vi "Simultaneous generation of analog voltage and digital signals.vi"() -> ()   [LabVIEW 2023]
uses:
  <vilib>/Utility/error.llb/DialogType.ctl
  <vilib>/DAQmx/configure/timing.llb/DAQmx Timing (Sample Clock).vi
  <vilib>/DAQmx/miscellaneous.llb/DAQmx Fill In Error Info.vi
  <vilib>/Waveform/DWDTOps.llb/DWDT Uncompress Digital.vi
  <vilib>/DAQmx/configure/trigger.llb/DAQmx Start Trigger (Digital Edge).vi
  <vilib>/DAQmx/create/channels.llb/DAQmx Create Channel (CO-Pulse Generation-Time).vi
  <vilib>/DAQmx/write.llb/DAQmx Write (Digital 1D Wfm NChan NSamp).vi
  <vilib>/DAQmx/create/channels.llb/DAQmx Create Channel (DO-Digital Output).vi
  <vilib>/DAQmx/write.llb/DAQmx Write (Analog 1D Wfm NChan NSamp).vi
  <vilib>/Waveform/DWDTOps.llb/DWDT Analog to Digital.vi
  <vilib>/DAQmx/create/channels.llb/DAQmx Create Channel (AO-Voltage-Basic).vi
  <resource>/objmgr/daqmx.rc
  <vilib>/measure/NI_MABase.lvlib
panel:
  in  "% of the time LEDs are shining\n(100 % maximum)":u32
  in  "Digital Channels for trigerring":tag
  out "Digital Waveform Graph":digitalwaveform[](graph)
  out "Waveform Graph":waveform(dbl)[](graph)
  in  "Stop Generation":bool caption="Stop Waveform Generation"
  in  "Analog Output Channels":tag
  out "Actual Duty Cycle (%)":dbl
  in  "Duty Cycle (%)":dbl
  in  "Square Wave Frequency (Hz)":dbl
  in  "LED Bias Voltage (V)":dbl[](array[numeric])
  # "AO0"
  # "AO1"
  # "AO2"
  # "AO3"
  # "If the duty cycle is set to 0, the default duty cycle will be applied, which depends on the number of channels active. 2 channels -> 50 %, 3 channels -> 33.33 %, 4 channels -> 25 %."
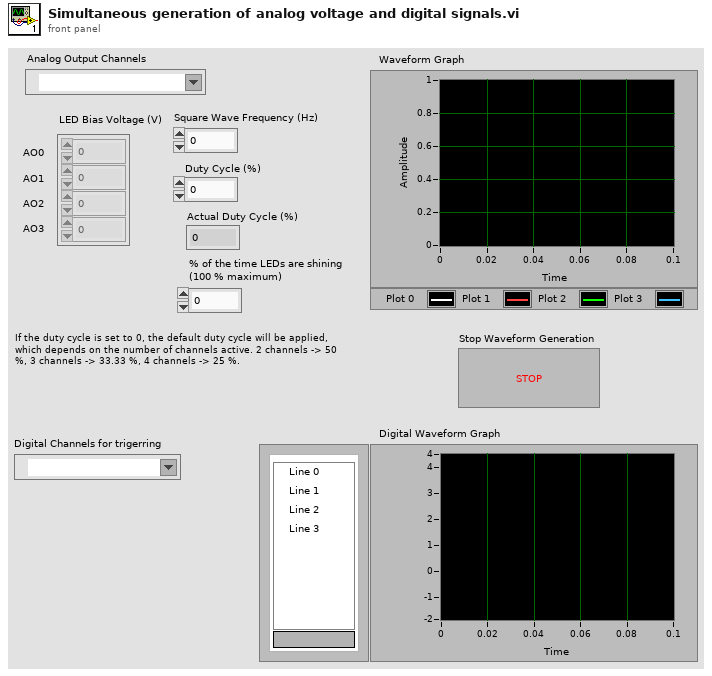
[diagram p1: front panel]
types:
  T1 = typedef "DialogType.ctl" = u16
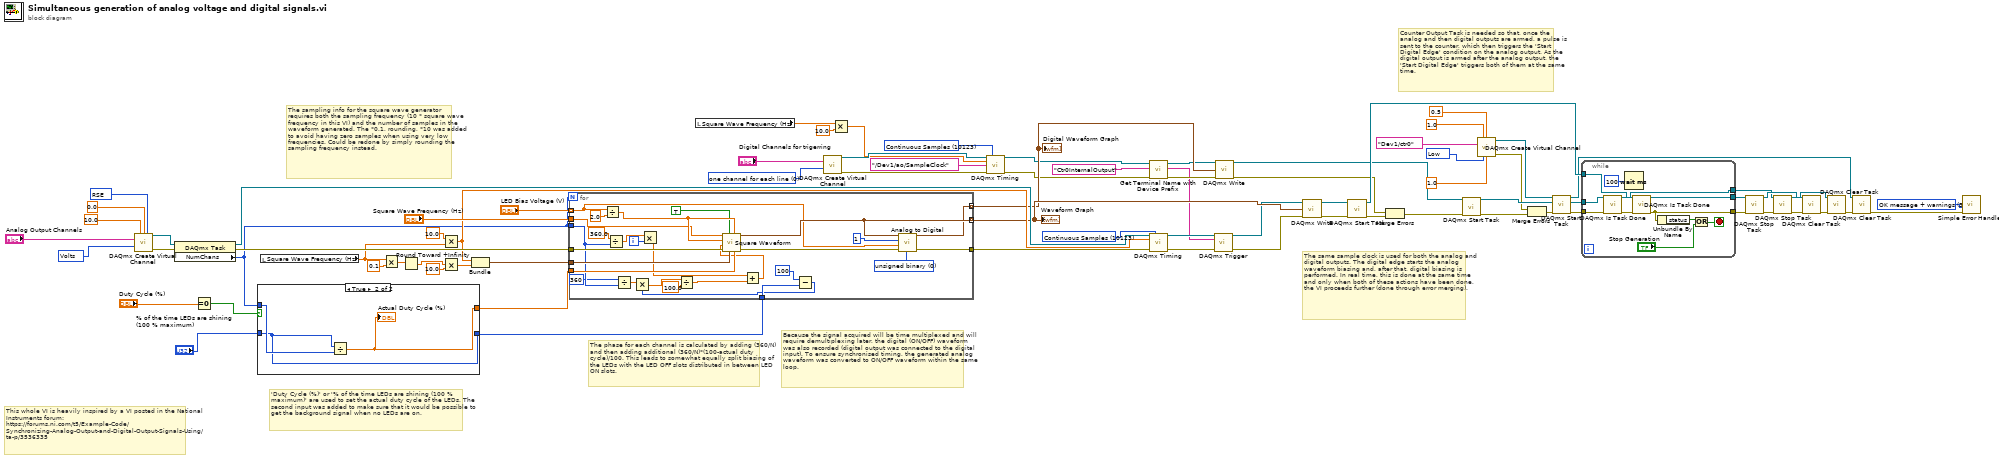
[diagram p0: block diagram]
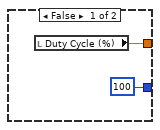
[diagram p2: hidden frame]
diagram:
  w24 = 10214 items=["High"=10192, "Low"=10214] ("idle state")
  w28 = 0 items=["one channel for each line", "one channel for all lines"] ("line grouping")
  w46 = 10123 items=["Finite Samples"=10178, "Continuous Samples"=10123, "Hardware Timed Single Point"=12522] ("sample mode")
  w52 = T1 3 items=["no dialog", "OK message", "continue or stop message", "OK message + warnings", "continue/stop + warnings"] ("type of dialog (OK msg:1)")
  w60 = 10123 items=["Finite Samples"=10178, "Continuous Samples"=10123, "Hardware Timed Single Point"=12522] ("sample mode")
  w77 = 10083 items=["Default"=-1, "RSE"=10083, "Differential"=10106, "Pseudodifferential"=12529] ("output terminal configuration")
  w78 = 10348 items=["Volts"=10348, "From Custom Scale"=10065] ("units")
  # "This whole VI is heavily inspired by a VI posted in the National Instruments forum:\nhttps://forums.ni.com/t5/Example-Code/Synchronizing-Analog-Output-and-Digital-Output-Signals-Using/ta-p/3536335"
  # "Counter Output Task is needed so that, once the analog and then digital outputs are armed, a pulse is sent to the counter, which then triggers the 'Start Digital Edge' condition on the analog output. As the digital output is armed after the analog output, the 'Start Digital Edge' triggers both of them at the same time."
  # "The same sample clock is used for both the analog and digital outputs. The digital edge starts the analog waveform biasing and, after that, digital biasing is performed. In real time, this is done at the same time and only when both of these actions have been done, the VI proceeds further (done through error merging)."
  # "Because the signal acquired will be time multiplexed and will require demultiplexing later, the digital (ON/OFF) waveform was also recorded (digital output was connected to the digital input). To ensure synchronised timing, the generated analog waveform was converted to ON/OFF waveform within the same loop."
  # "The phase for each channel is calculated by adding (360/N) and then adding additional (360/N)*(100-actual duty cycle)/100. This leads to somewhat equally split biasing of the LEDs with the LED OFF slots distributed in between LED ON slots."
  # "The sampling info for the square wave generator requires both the sampling frequency (10 * square wave frequency in this VI) and the number of samples in the waveform generated. The *0.1, rounding, *10 was added to avoid having zero samples when using very low frequencies. Could be redone by simply rounding the sampling frequency instead."
  # "'Duty Cycle (%)' or '% of the time LEDs are shining (100 % maximum)' are used to set the actual duty cycle of the LEDs. The second input was added to make sure that it would be possible to get the background signal when no LEDs are on."
  n1 = call-poly <vilib>:"DAQmx Create Virtual Channel.vi"("maximum value"=10.0, "minimum value"=0.0, "output terminal configuration"=w77, "physical channels"="Analog Output Channels", "units"=w78) -> ("task out"=w74:refnum<k21>, "error out"=w73:errorcluster)  [unwired: 9 in]
  n2 = property class="DAQmx Task"(reference=w74, error in=w73) -> (reference out=w58:refnum<k21>, error out=w70:errorcluster, "NumChans"=w48:u32)
  n3 = Equal To 0?(x="Duty Cycle (%)") -> (x = 0?=w68:bool)
  n4 = case shown="True" w68 {
    tunnel: [w81 w83] -> w67
    tunnel: w48 -> [_ w84]
    tunnel: [u32 100 ("% of the time LEDs are shining\n(100 % maximum)") w82] -> w4
    tunnel: "% of the time LEDs are shining\n(100 % maximum)" -> [_ w82]
    frame False {
      n5 = local read "Duty Cycle (%)"() -> (w81:dbl)
    }
    frame True {
      n6 = Divide(x=w82, y=w84) -> (x/y=w83:dbl)
      "Actual Duty Cycle (%)" <- w83
    }
  }
  n7 = local read "Square Wave Frequency (Hz)"() -> (w62:dbl)
  n8 = Multiply(x=w62, y=0.1) -> (x*y=w2:dbl)
  n9 = Round Toward +Infinity(x=w2) -> (ceil(x): smallest int >= x=w1:dbl)
  n10 = Multiply(x=10.0, y=w62) -> (x*y=w57:dbl)
  n11 = Multiply(x=w1, y=10.0) -> (x*y=w64:dbl)
  n12 = Bundle(w57, w64) -> (w61:cluster{dbl, dbl})  [unwired: 1 in]
  n13 = for {
    N: w48 -> [_]
    tunnel: "LED Bias Voltage (V)" -> [w101] mode=indexing
    tunnel: "Square Wave Frequency (Hz)" -> [w110]
    tunnel: w70 -> [w109]
    tunnel: w67 -> [w108]
    tunnel: w61 -> [w107]
    tunnel: [w98] -> w59
    tunnel: [w102] -> w49 mode=indexing
    tunnel: w48 -> [w94]
    tunnel: [w100] -> w39 mode=indexing
    tunnel: w4 -> [w92]
    i -> [w104]
    w96 = u16 0 items=["unsigned binary", "offset binary", "2's complement"] ("data format (offset binary)")
    n14 = Divide(x=w101, y=2.0) -> (x/y=w111:dbl)
    n15 = Divide(x=360.0, y=w94) -> (x/y=w103:dbl)
    n16 = Divide(x=u32 360, y=w94) -> (x/y=w90:dbl)
    n17 = Multiply(x=w103, y=w104) -> (x*y=w95:dbl)
    n18 = Subtract(x=u32 100, y=w92) -> (x-y=w89:u32)
    n19 = Multiply(x=w90, y=w89) -> (x*y=w88:dbl)
    n20 = Divide(x=w88, y=100.0) -> (x/y=w86:dbl)
    n21 = Add(x=w95, y=w86) -> (x+y=w85:dbl)
    n22 = call <vilib>:"Square Waveform.vi"("duty cycle (%)"=w108, "offset"=w111, "sampling info"=w107, "reset signal"=TRUE, "error in (no error)"=w109, "phase"=w85, "amplitude"=w111, "frequency"=w110) -> ("error out"=w99:errorcluster, "signal out"=w102:waveform(dbl))  [unwired: 2 in]
    n23 = call-poly <vilib>:"Analog to Digital.vi"("data format (offset binary)"=w96, "error in (no error)"=w99, "full-scale range (pk-pk)"=w101, "resolution (16 bit)"=1, "analog waveform"=w102) -> ("error out"=w98:errorcluster, "digital waveform"=w100:digitalwaveform)  [unwired: 3 in, 2 out]
  }
  "Waveform Graph" <- w49
  "Digital Waveform Graph" <- w39
  n24 = local read "Square Wave Frequency (Hz)"() -> (w43:dbl)
  n25 = call-poly <vilib>:"DAQmx Create Virtual Channel.vi"("lines"="Digital Channels for trigerring", "line grouping"=w28) -> ("task out"=w44:refnum<k21>, "error out"=w45:errorcluster)  [unwired: 12 in]
  n26 = Multiply(x=w43, y=10.0) -> (x*y=w41:dbl)
  n27 = call-poly <vilib>:"DAQmx Timing.vi"("task/channels in"=w44, "sample mode"=w46, "rate"=w41, "source"=tag "/Dev1/ao/SampleClock", "error in"=w45) -> ("task out"=w22:refnum<k21>, "error out"=w21:errorcluster)  [unwired: 9 in]
  n28 = call "Get Terminal Name with Device Prefix.vi"("error in (no error)"=w21, "Local Terminal Name"="Ctr0InternalOutput", "task/channels in"=w22) -> ("error out"=w19:errorcluster, "Terminal Name with Device Prefix"=w13:tag, "task out"=w20:refnum<k21>)  [unwired: 6 in]
  n29 = call-poly <vilib>:"DAQmx Timing.vi"("task/channels in"=w58, "sample mode"=w60, "rate"=w57, "error in"=w59) -> ("task out"=w16:refnum<k21>, "error out"=w17:errorcluster)  [unwired: 10 in]
  n30 = call-poly <vilib>:"DAQmx Trigger.vi"("task/channels in"=w16, "source"=w13, "error in"=w17) -> ("task out"=w14:refnum<k21>, "error out"=w15:errorcluster)  [unwired: 11 in]
  n31 = call-poly <vilib>:"DAQmx Write.vi"("task/channels in"=w20, "data"=w39, "error in"=w19) -> ("task out"=w36:refnum<k21>, "error out"=w37:errorcluster)  [unwired: 10 in, 1 out]
  n32 = call-poly <vilib>:"DAQmx Write.vi"("task/channels in"=w14, "data"=w49, "error in"=w15) -> ("task out"=w56:refnum<k21>, "error out"=w55:errorcluster)  [unwired: 10 in, 1 out]
  n33 = call <vilib>:"DAQmx Start Task.vi"("task/channels in"=w56, "error in"=w55) -> ("task out"=w54:refnum<k21>, "error out"=w38:errorcluster)  [unwired: 12 in]
  n34 = Merge Errors(w37, w38) -> (w35:errorcluster)
  n35 = call <vilib>:"DAQmx Start Task.vi"("task/channels in"=w36, "error in"=w35) -> ("task out"=w34:refnum<k21>, "error out"=w12:errorcluster)  [unwired: 12 in]
  n36 = call-poly <vilib>:"DAQmx Create Virtual Channel.vi"("high time"=1.0, "low time"=0.5, "counter"=tag "Dev1/ctr0", "idle state"=w24, "initial delay"=1.0) -> ("task out"=w9:refnum<k21>, "error out"=w11:errorcluster)  [unwired: 9 in]
  n37 = Merge Errors(w11, w12) -> (w10:errorcluster)
  n38 = call <vilib>:"DAQmx Start Task.vi"("task/channels in"=w9, "error in"=w10) -> ("task out"=w7:refnum<k21>, "error out"=w8:errorcluster)  [unwired: 12 in]
  n39 = while {
    tunnel: w54 -> [w123]
    tunnel: [w117] -> w51
    tunnel: [w118] -> w50
    tunnel: w34 -> [w116]
    tunnel: w8 -> [w115]
    tunnel: [w113] -> w33
    stop <- w121 stop-if-true
    n40 = call <vilib>:"DAQmx Is Task Done.vi"("task/channels in"=w116, "error in"=w115) -> ("task out"=w113:refnum<k21>, "error out"=w114:errorcluster)  [unwired: 11 in, 1 out]
    n41 = Wait (ms)(milliseconds to wait=u32 100) -> ()  [unwired: 1 out]
    n42 = call <vilib>:"DAQmx Is Task Done.vi"("task/channels in"=w123, "error in"=w114) -> ("task out"=w118:refnum<k21>, "error out"=w117:errorcluster)  [unwired: 11 in, 1 out]
    n43 = Unbundle By Name(w117) -> ("status"=w119:bool)
    n44 = Or(x=w119, y="Stop Generation") -> (x .or. y?=w121:bool)
  }
  n45 = call <vilib>:"DAQmx Stop Task.vi"("task/channels in"=w50, "error in"=w51) -> ("task out"=w53:refnum<k21>, "error out"=w32:errorcluster)  [unwired: 12 in]
  n46 = call <vilib>:"DAQmx Stop Task.vi"("task/channels in"=w33, "error in"=w32) -> ("task out"=w30:refnum<k21>, "error out"=w31:errorcluster)  [unwired: 12 in]
  n47 = call <vilib>:"DAQmx Clear Task.vi"("task in"=w53, "error in"=w31) -> ("error out"=w29:errorcluster)  [unwired: 13 in]
  n48 = call <vilib>:"DAQmx Clear Task.vi"("task in"=w30, "error in"=w29) -> ("error out"=w6:errorcluster)  [unwired: 13 in]
  n49 = call <vilib>:"DAQmx Clear Task.vi"("task in"=w7, "error in"=w6) -> ("error out"=w5:errorcluster)  [unwired: 13 in]
  n50 = call <vilib>:"Simple Error Handler.vi"("type of dialog (OK msg:1)"=w52, "error in (no error)"=w5) -> ()  [unwired: 3 in, 5 out]
